vi "CFTS-Aborted Run File Save Query.vi"(0 "Expt State":T2, 5 "Path":path, 7 "Aborted":bool, 11 "error in (no error)":errorcluster, 12 "Data Type":T1) -> (4 "Expt State out":T2, 8 "File saved?":bool, 15 "error out":errorcluster)   [LabVIEW 2020]
uses:
  CFTS-Experiment State.ctl
  CFTS-Data Type Enum.ctl
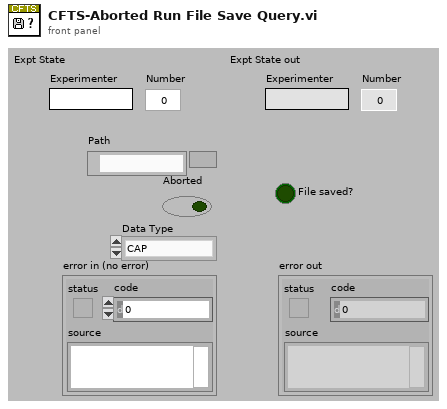
[diagram p1: front panel]
types:
  T1 = typedef "CFTS-Data Type Enum.ctl" = enum16{"CAP", "ABR", "DP", "VsEP", "MeasSeq", "SFOAE"}
  T2 = typedef "CFTS-Experiment State.ctl" = cluster{"Experimenter":string, "Number":u32, "Right":string, "Left":string, "Data Folder":path, "State File":path, "Version Info":string, "End Exposure Time":dbl, "Exposure Duration":string, "Run #":cluster{"CAP":i16, "ABR":i16, "DP":i16, "VsEP":i16, "MeasSeq":i16, "SubSeq":i16, "SFOAE":i16}}
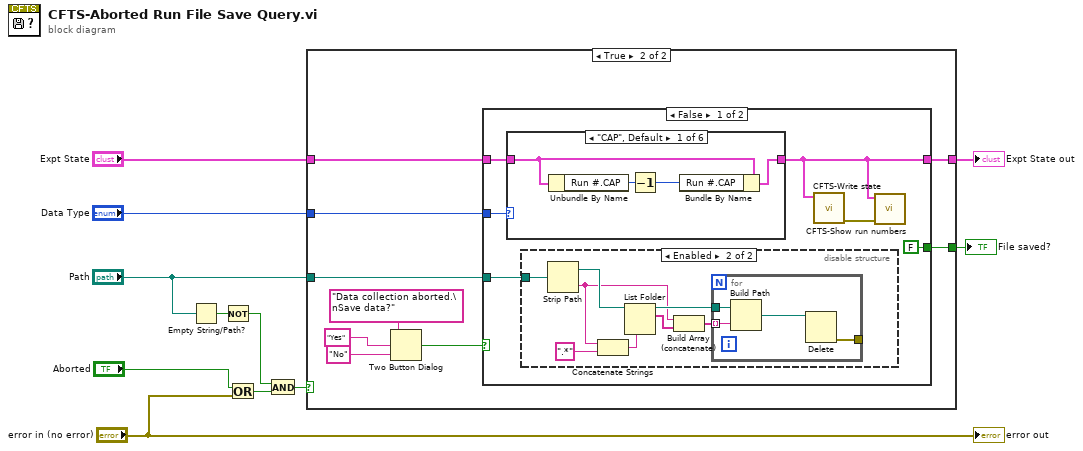
[diagram p0: block diagram]
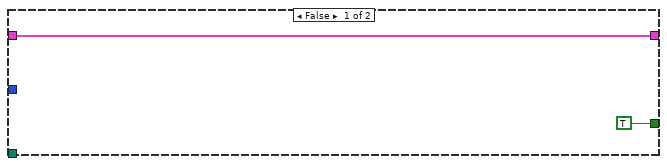
[diagram p2: hidden frame]
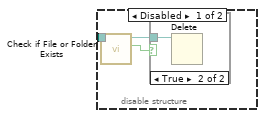
[diagram p3: hidden frame]
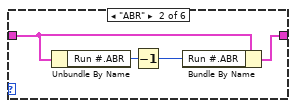
[diagram p5: hidden frame]
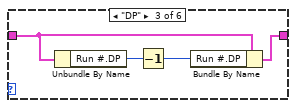
[diagram p6: hidden frame]
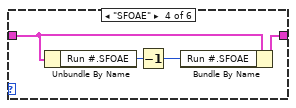
[diagram p7: hidden frame]
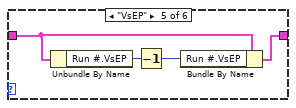
[diagram p8: hidden frame]
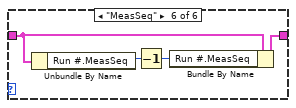
[diagram p9: hidden frame]
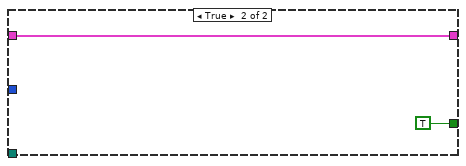
[diagram p10: hidden frame]
diagram:
  n1 = Empty String/Path?(string/path="Path") -> (empty?=w3:bool)
  n2 = Not(x=w3) -> (.not. x?=w2:bool)
  n3 = Or(x="Aborted", y="error in (no error)") -> (x .or. y?=w10:bool)
  n4 = And(x=w2, y=w10) -> (x .and. y?=w5:bool)
  n5 = case shown="True" w5 {
    tunnel: "Path" -> [_ w18]
    tunnel: "Data Type" -> [_ w17]
    tunnel: "Expt State" -> [w13 w16]
    tunnel: [w13 w15] -> w7
    tunnel: [TRUE w14] -> w6
    frame False {
    }
    frame True {
      n6 = Two Button Dialog(message="Data collection aborted.\nSave data?", 1:"No" ("F button name (\"Cancel\")"), 2:"Yes" ("T button name (\"OK\")")) -> (T button?=w19:bool)
      n7 = case shown="False" w19 {
        tunnel: w18 -> [w23 _]
        tunnel: w17 -> [w28 _]
        tunnel: w16 -> [w27 w70]
        tunnel: [w25 w70] -> w15
        tunnel: [FALSE TRUE] -> w14
        frame False {
          n8 = case shown="\"CAP\", Default" w28 {
            tunnel: w27 -> [w48 w52 w56 w60 w64 w68]
            tunnel: [w46 w50 w54 w58 w62 w66] -> w25
            frame "CAP", Default {
              n9 = Unbundle By Name(w48) -> ("Run #.CAP"=w47:i16)
              n10 = Decrement(x=w47) -> (x-1=w45:i16)
              n11 = Bundle By Name(cluster=w48, "Run #.CAP"=w45) -> (w46:T2)
            }
            frame "ABR" {
              n12 = Unbundle By Name(w52) -> ("Run #.ABR"=w51:i16)
              n13 = Decrement(x=w51) -> (x-1=w49:i16)
              n14 = Bundle By Name(cluster=w52, "Run #.ABR"=w49) -> (w50:T2)
            }
            frame "DP" {
              n15 = Unbundle By Name(w56) -> ("Run #.DP"=w55:i16)
              n16 = Decrement(x=w55) -> (x-1=w53:i16)
              n17 = Bundle By Name(cluster=w56, "Run #.DP"=w53) -> (w54:T2)
            }
            frame "SFOAE" {
              n18 = Unbundle By Name(w60) -> ("Run #.SFOAE"=w59:i16)
              n19 = Decrement(x=w59) -> (x-1=w57:i16)
              n20 = Bundle By Name(cluster=w60, "Run #.SFOAE"=w57) -> (w58:T2)
            }
            frame "VsEP" {
              n21 = Unbundle By Name(w64) -> ("Run #.VsEP"=w63:i16)
              n22 = Decrement(x=w63) -> (x-1=w61:i16)
              n23 = Bundle By Name(cluster=w64, "Run #.VsEP"=w61) -> (w62:T2)
            }
            frame "MeasSeq" {
              n24 = Unbundle By Name(w68) -> ("Run #.MeasSeq"=w67:i16)
              n25 = Decrement(x=w67) -> (x-1=w65:i16)
              n26 = Bundle By Name(cluster=w68, "Run #.MeasSeq"=w65) -> (w66:T2)
            }
          }
          n27 = disable-structure shown="Enabled" {
            disable-tunnel: w23 -> [w29 w37]
            frame Disabled {
              n28 = call <vilib>:"Check if File or Folder Exists.vi"("path"=w29) -> ("file or folder exists?"=w30:bool, "dup path"=w31:path)  [unwired: 8 in, 1 out]
              n29 = case shown="True" w30 {
                tunnel: w31 -> [_ w32]
                frame False {
                }
                frame True {
                  n30 = Delete(path (use dialog)=w32) -> ()  [unwired: 4 in, 3 out]
                }
              }
            }
            frame Enabled {
              n31 = Strip Path(path=w37) -> (stripped path=w40:path, name=w33:string)
              n32 = Concatenate Strings(w33, ".*" ("string")) -> (w38:string)
              n33 = List Folder(path=w40, pattern=w38) -> (path out=w36:path, filenames=w35:string[])  [unwired: 2 in, 2 out]
              n34 = Build Array (concatenate)(w33, w35) -> (w34:string[])
              n35 = for {
                tunnel: w36 -> [w44]
                tunnel: w34 -> [w42] mode=indexing
                tunnel: [w41] -> _
                n36 = Build Path(base path=w44, name or relative path=w42) -> (appended path=w43:path)
                n37 = Delete(path (use dialog)=w43) -> (error out=w41:errorcluster)  [unwired: 4 in, 2 out]
              }
            }
          }
          n38 = call "CFTS-Write state.vi"("Experiment info"=w25) -> ("error out"=w26:errorcluster)  [unwired: 10 in]
          n39 = call "CFTS-Show run numbers.vi"("error in (no error)"=w26, "Expt State"=w25) -> ()  [unwired: 9 in, 1 out]
        }
        frame True {
        }
      }
    }
  }
  "Expt State out" <- w7
  "File saved?" <- w6
  "error out" <- "error in (no error)"
